vi "Close FileTx Notifier.vi"(8 "error in (no error)":errorcluster, 11 "FTP in":refnum<class "FTP.lvclass">) -> (0 "error out":errorcluster, 3 "FTP out":refnum<class "FTP.lvclass">)   [LabVIEW 2017, in "FTP_UpgradeCSMF.lvlib" / "FTP.lvclass"]
uses:
  FTP.lvclass
  controls/File Transfer Status.ctl
  FTP.lvclass/FTP.ctl
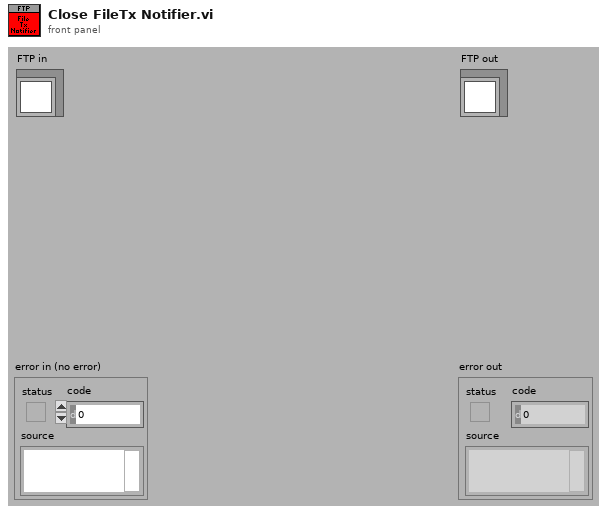
[diagram p1: front panel]
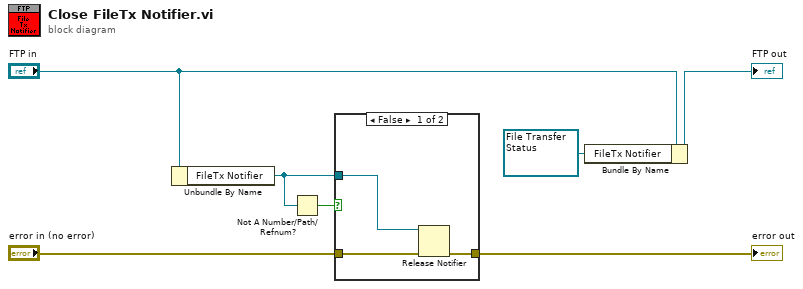
[diagram p0: block diagram]
diagram:
  n1 = Unbundle By Name("FTP in") -> ("FileTx Notifier"=w3:refnum<notifier>)
  n2 = Not A Number/Path/Refnum?(number/path/refnum=w3) -> (NaN/Path/Refnum?=w2:bool)
  n3 = case shown="False" w2 {
    tunnel: w3 -> [w10 _]
    tunnel: "error in (no error)" -> [w9 w11]
    tunnel: [w8 w11] -> w6
    frame False {
      n4 = Release Notifier(notifier=w10, error in (no error)=w9) -> (error out=w8:errorcluster)  [unwired: 1 in, 2 out]
    }
    frame True {
    }
  }
  "error out" <- w6
  n5 = Bundle By Name(cluster="FTP in", "FileTx Notifier"=refnum<notifier> refnum) -> (→"FTP out":refnum<class "FTP.lvclass">)
